vi "Assemble Splash Screen ViewManager.vi"(10 "Process Builder ViewManager":refnum<class "Navigation ViewManager.lvclass">, 11 "Loading View":refnum<class "Loading View.lvclass">) -> (3 "Splash Screen ViewManager out":refnum<class "Splash Screen ViewManager.lvclass">)   [LabVIEW 2019, in "Splash Screen ViewManager.lvclass"]
uses:
  <vilib>/gpm_packages/@cs/Car-wash/Source/Splash Screen ViewManager/Splash Screen ViewManager.lvclass
  C:/Program Files/National Instruments/LabVIEW 2019/vi.lib/gpm_packages/@cs/mva-viewable/Source/IViewManager/IViewManager/IViewManager.lvclass
  <vilib>/gpm_packages/@cs/Car-wash/Source/Loading View/Loading View.lvclass
  C:/Program Files/National Instruments/LabVIEW 2019/vi.lib/gpm_packages/@cs/mva-viewable/Source/IViewable/IViewable/IViewable.lvclass
  <vilib>/gpm_packages/@cs/Car-wash/Source/Process Builder ViewManager/Navigation ViewManager.lvclass
  <vilib>/gpm_packages/@cs/mva-viewable/Source/IViewManager/IViewManager Messages/Launch Nested Views Msg/Launch Nested Views Msg.lvclass/Launch Nested Views Msg.ctl
  <vilib>/gpm_packages/@cs/mva-viewable/Source/IViewManager/IViewManager/IViewManager.lvclass/IViewManager.ctl
  <vilib>/gpm_packages/@cs/mva-viewable/Source/IViewManager/IViewManager Messages/Launch Nested Views Msg/Pack Launch Nested Views Msg.vi
  <vilib>/gpm_packages/@cs/mva-viewable/Source/IViewManager/IViewManager Messages/Launch Nested Views Msg/Launch Nested Views Msg.lvclass
  <vilib>/gpm_packages/@cs/mva-viewable/Source/IViewManager/IViewManager/IViewManager.lvclass
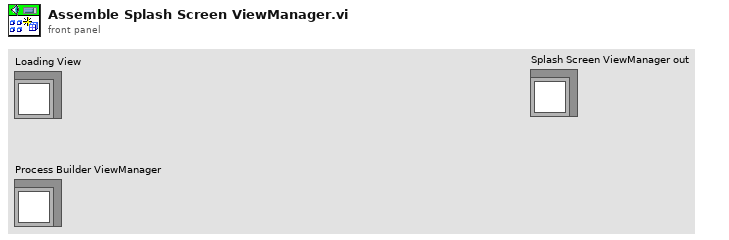
[diagram p1: front panel]
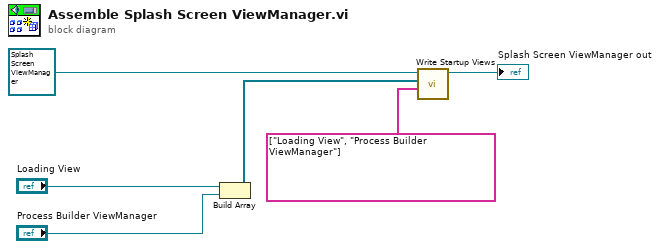
[diagram p0: block diagram]
diagram:
  n1 = Build Array("Loading View", "Process Builder ViewManager") -> (w4:refnum<class "IViewable.lvclass">[])
  n2 = call <vilib>:"Write Startup Views.vi"("View Labels"=string[] ["Loading View", "Process Builder ViewManager"], "Startup Views"=w4, "IViewManager in"=refnum<class "Splash Screen ViewManager.lvclass"> refnum ("Main ViewManager.lvlib:Main ViewManager.lvclass")) -> ("IViewManager out"=→"Splash Screen ViewManager out":refnum<class "Splash Screen ViewManager.lvclass">)  [unwired: 8 in]
